vi "Get ID.vi"(8 "error in (no error)":errorcluster, 11 "PS_Sim in":refnum<class "PS Simulated.lvclass">) -> (0 "error out":errorcluster, 3 "PS_Sim out":refnum<class "PS Simulated.lvclass">)   [LabVIEW 2021, in "PS.lvlib" / "PS Simulated.lvclass"]
uses:
  PS Simulated.lvclass
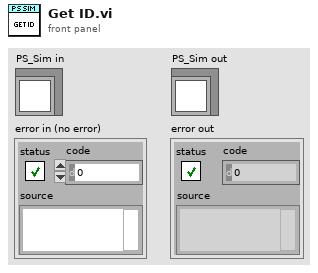
[diagram p1: front panel]
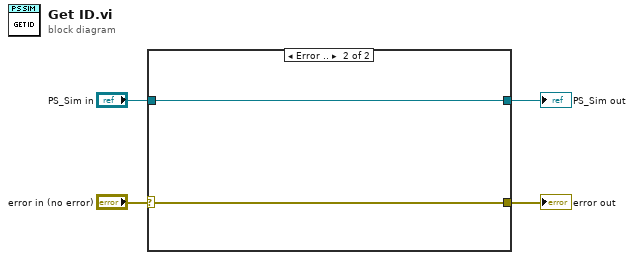
[diagram p0: block diagram]
diagram:
  n1 = case shown="Error .." "error in (no error)" {
    selector: "error in (no error)" -> [w5 w7]
    tunnel: [w6 w8] -> w3
    tunnel: "PS_Sim in" -> [w6 w8]
    tunnel: [w5 w7] -> w1
    frame No Error {
    }
    frame Error {
    }
  }
  "error out" <- w1
  "PS_Sim out" <- w3
